vi "Run Infuse.vi"(7 "auto_switch_valve":bool=TRUE, 8 "error in (no error)":errorcluster, 9 "Flow rate, uL/s":dbl=25.0, 10 "Volume, uL":dbl=100.0, 11 "PHD Ultra in":refnum<class "PHD Ultra.lvclass">) -> (0 "error out":errorcluster, 3 "PHD Ultra out":refnum<class "PHD Ultra.lvclass">)   [LabVIEW 2018, in "PHD Ultra.lvlib" / "PHD Ultra.lvclass"]
uses:
  PHD Ultra.lvclass
  <userlib>/QmixLib/QmixLib.lvlib
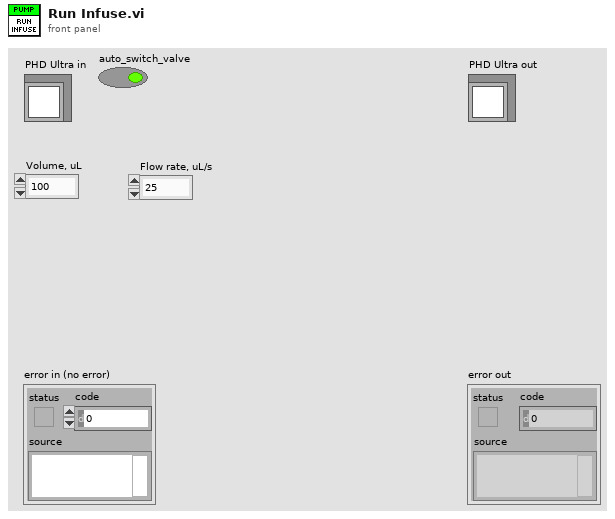
[diagram p1: front panel]
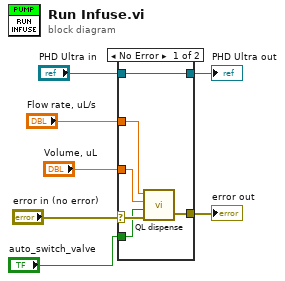
[diagram p0: block diagram]
diagram:
  n1 = case shown="No Error" "error in (no error)" {
    selector: "error in (no error)" -> [w11 w15]
    tunnel: [w12 w15] -> w6
    tunnel: [w13 w14] -> w4
    tunnel: "PHD Ultra in" -> [w13 w14]
    tunnel: "Volume, uL" -> [w10 _]
    tunnel: "Flow rate, uL/s" -> [w9 _]
    tunnel: "auto_switch_valve" -> [w8 _]
    frame No Error {
      n2 = call <userlib>:"QL dispense.vi"("error in (no error)"=w11, "auto_switch_valve"=w8, "volume_uL"=w10, "flow_rate_uL_s"=w9) -> ("error out"=w12:errorcluster)  [unwired: 3 in]
    }
    frame Error {
    }
  }
  "error out" <- w6
  "PHD Ultra out" <- w4
